vi "Check_In_Range.vi"(8 "error in (no error)":errorcluster, 10 "channel name":string, 11 "instrument handle":refnum<k15>) -> (0 "error out":errorcluster, 3 "not in compliance?":bool=TRUE)   [LabVIEW 2021, in "niDCPower.lvclass"]
uses:
  niDCPower.lvclass
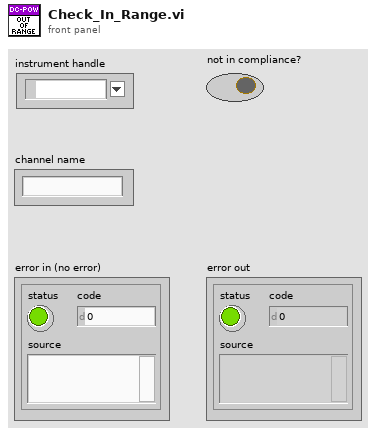
[diagram p1: front panel]
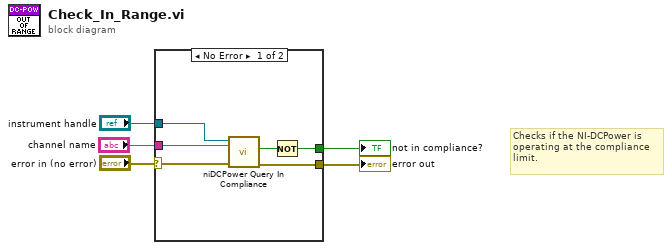
[diagram p0: block diagram]
diagram:
  # "Checks if the NI-DCPower is\noperating at the compliance\nlimit."
  n1 = case shown="No Error" "error in (no error)" {
    selector: "error in (no error)" -> [w10 w12]
    tunnel: "instrument handle" -> [w11 _]
    tunnel: "channel name" -> [w9 _]
    tunnel: [w8 w12] -> w2
    tunnel: [w6 _] -> w1
    frame No Error {
      n2 = call <instrlib>:"niDCPower Query In Compliance.vi"("error in (no error)"=w10, "channel name"=w9, "instrument handle"=w11) -> ("error out"=w8:errorcluster, "in compliance?"=w7:bool)  [unwired: 6 in, 1 out]
      n3 = Not(x=w7) -> (.not. x?=w6:bool)
    }
    frame Error {
    }
  }
  "error out" <- w2
  "not in compliance?" <- w1
